vi "Trigger Circuitry (U8).vi"(6 "SM Ready for Trigger":bool, 7 "Trigger Type":T2(ring)=enum."Software Trigger", 8 "Input Valid":bool, 9 "Analog Trigger Setup":T1, 10 "Digital Trigger Value":u8, 11 "Software Trigger from Host":bool) -> (0 "Output Valid":bool, 2 "Trigger Out":bool, 3 "Analog Arm Trig":bool, 4 "Trig Offset":u8)   [LabVIEW 2012]
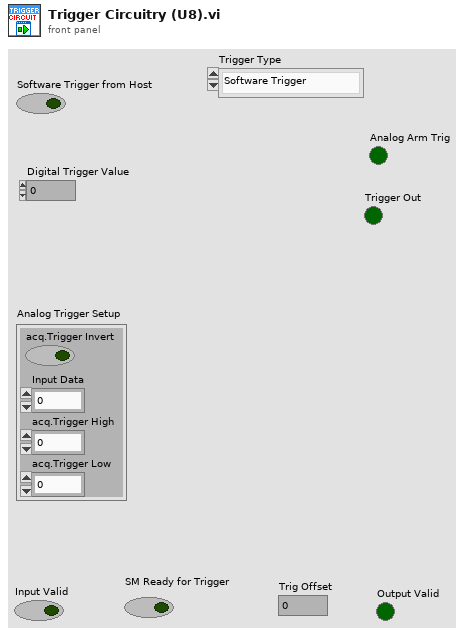
[diagram p1: front panel]
types:
  T1 = cluster{"acq.Trigger Invert":bool, "Input Data":i16, "acq.Trigger High":i16, "acq.Trigger Low":i16}
  T2 = enum8{"Immediate Trigger", "Software Trigger", "External Digital Trigger", "Analog Trigger"}
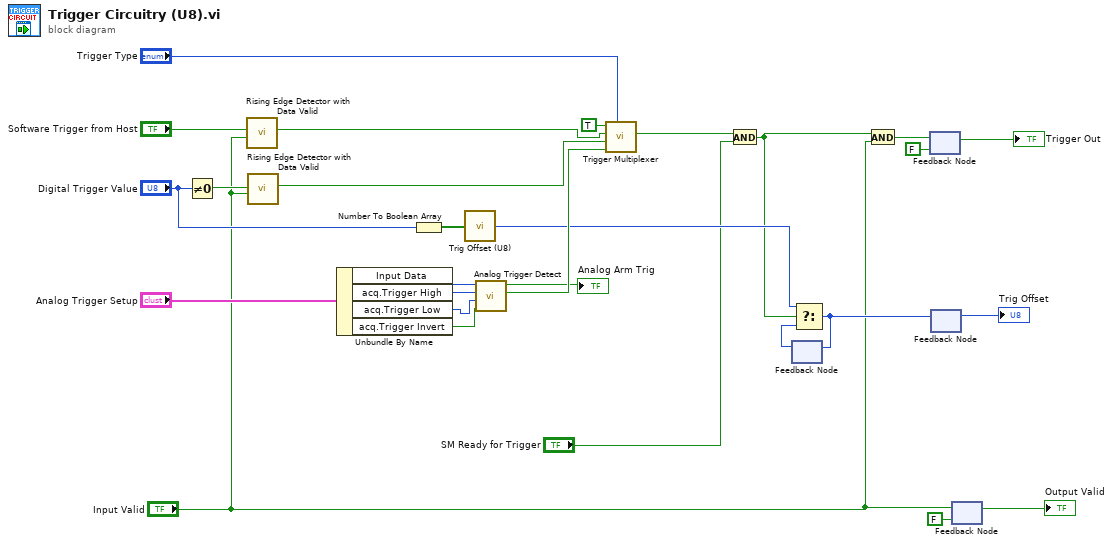
[diagram p0: block diagram]
diagram:
  n1 = Not Equal To 0?(x="Digital Trigger Value") -> (x != 0?=w18:bool)
  n2 = call <userlib>:"Rising Edge Detector with Data Valid.vi"("Data Valid"="Input Valid", "signal"="Software Trigger from Host") -> ("edge detected"=w7:bool)  [unwired: 9 in]
  n3 = call <userlib>:"Rising Edge Detector with Data Valid.vi"("Data Valid"="Input Valid", "signal"=w18) -> ("edge detected"=w17:bool)  [unwired: 9 in]
  n4 = Unbundle By Name("Analog Trigger Setup") -> ("Input Data"=w23:i16, "acq.Trigger High"=w22:i16, "acq.Trigger Low"=w21:i16, "acq.Trigger Invert"=w20:bool)
  n5 = Number To Boolean Array(number="Digital Trigger Value") -> (Boolean array=w16:bool[])
  n6 = call <userlib>:"Trig Offset (U8).vi"("Trig Values [n-7] to n"=w16) -> ("Trigger Offset"=w14:u8)  [unwired: 14 in]
  n7 = call <userlib>:"Analog Trigger Detect.vi"("acq.Trigger Invert"=w20, "acq.Trigger High"=w21, "acq.Trigger Low"=w22, "Input Data"=w23) -> ("Analog Trigger Detect"=w28:bool, "Analog Arm Trig"=→"Analog Arm Trig":bool)  [unwired: 6 in]
  n8 = call <userlib>:"Trigger Multiplexer.vi"("Trigger Type"="Trigger Type", "Analog Trigger"=w28, "Digital Trigger"=w17, "Software Trigger"=w7, "Immediate Trigger"=TRUE) -> ("Trigger Out"=w2:bool)  [unwired: 6 in]
  n9 = And(x=w2, y="SM Ready for Trigger") -> (x .and. y?=w1:bool)
  n10 = feedback #1() -> (w15:u8)  [unwired: 1 in]
  n11 = Select(t=w14, s=w1, f=w15) -> (s? t:f=w13:u8)
  n12 = feedback-in #1(w13) -> ()
  n13 = And(x=w1, y="Input Valid") -> (x .and. y?=w8:bool)
  n14 = feedback-in #2(w8) -> ()
  n15 = feedback #2(FALSE) -> (→"Trigger Out":bool)
  n16 = feedback-in #3(w13) -> ()
  n17 = feedback #3() -> (→"Trig Offset":u8)  [unwired: 1 in]
  n18 = feedback-in #4("Input Valid") -> ()
  n19 = feedback #4(FALSE ("Input Valid")) -> (→"Output Valid":bool)
